vi "CAN_Init.vi"(0 "object in":refnum<class "NI-XNET.lvclass">, 5 "CAN Init Data":T1={"XNET Interface"="", "Baud Rate"=500000, "CAN:Termination"=0, "Echo Transmit?"=FALSE, "scope (normal)"=1} {"scope (normal)" items=["Normal", "Session Only", "Interface Only", "Session Only Blocking"]; "CAN:Termination" items=["Off", "On"]; "Baud Rate" format="%.0p"}, 11 "error in (no error)":errorcluster) -> (4 "object out":refnum<class "NI-XNET.lvclass">, 15 "error out":errorcluster)   [LabVIEW 2023, in "HardwareAbstractionLayer_LVOOP.lvlib" / "CAN HAL Lib.lvlib" / "NI-XNET.lvclass"]
uses:
  NI-XNET.lvclass
  CAN_class/Ctrls/CAN Init Ctrl.ctl
  <vilib>/xnet/xnet.llb/XNET Control Scope.ctl
  NI-XNET.lvclass/NI-XNET.ctl
  CAN_class/CAN.lvclass
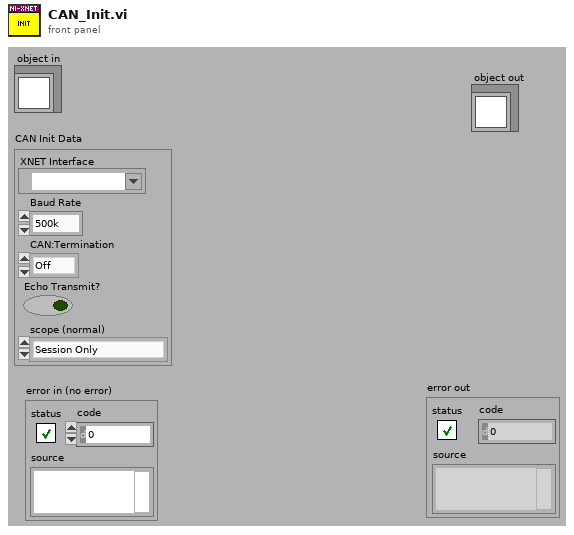
[diagram p1: front panel]
types:
  T1 = typedef "HardwareAbstractionLayer_LVOOP.lvlib/CAN HAL Lib.lvlib/CAN.lvclass/CAN Init Ctrl.ctl" = cluster{"XNET Interface":refnum<k21>, "Baud Rate":u64, "CAN:Termination":u32, "Echo Transmit?":bool, "scope (normal)":T2}
  T2 = typedef "XNET Control Scope.ctl" = u32
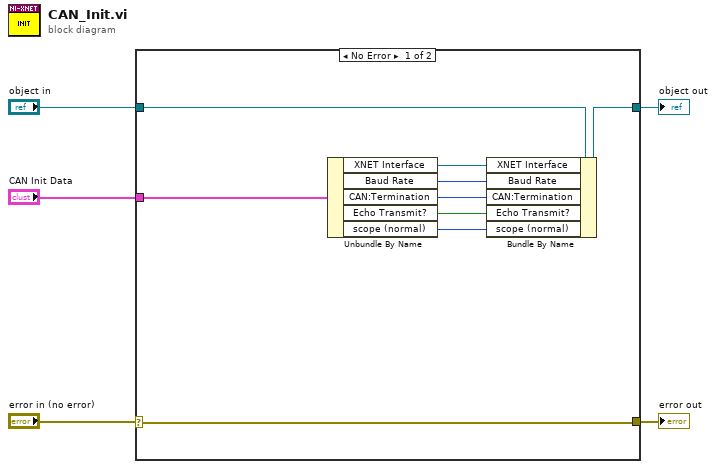
[diagram p0: block diagram]
diagram:
  n1 = case shown="No Error" "error in (no error)" {
    selector: "error in (no error)" -> [w11 w15]
    tunnel: [w14 w16] -> w5
    tunnel: "object in" -> [w13 w16]
    tunnel: [w11 w15] -> w2
    tunnel: "CAN Init Data" -> [w12 _]
    frame No Error {
      n2 = Unbundle By Name(w12) -> ("XNET Interface"=w10:refnum<k21>, "Baud Rate"=w9:u64, "CAN:Termination"=w8:u32, "Echo Transmit?"=w7:bool, "scope (normal)"=w6:T2)
      n3 = Bundle By Name(cluster=w13, "XNET Interface"=w10, "Baud Rate"=w9, "CAN:Termination"=w8, "Echo Transmit?"=w7, "scope (normal)"=w6) -> (w14:refnum<class "NI-XNET.lvclass">)
    }
    frame Error {
    }
  }
  "object out" <- w5
  "error out" <- w2
